vi "check_folder (SubVI).vi"(11 "path in":path) -> (3 "path out":path)   [LabVIEW 2014]
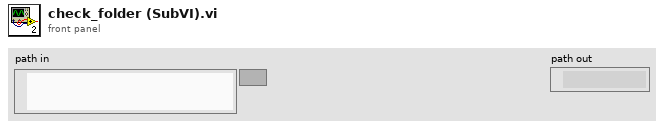
[diagram p1: front panel]
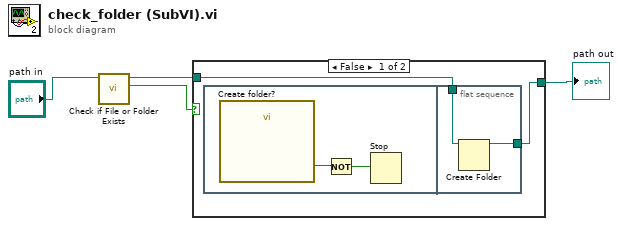
[diagram p0: block diagram]
diagram:
  n1 = call <vilib>:"Check if File or Folder Exists.vi"("path"="path in") -> ("file or folder exists?"=w3:bool, "dup path"=w4:path)  [unwired: 8 in, 1 out]
  n2 = case shown="False" w3 {
    tunnel: w4 -> [w6 w11]
    tunnel: [w5 w11] -> w1
    frame False {
      n3 = flat-sequence {
        tunnel: w6 -> [w10]
        tunnel: [w9] -> w5
        frame #0 {
          n4 = call "Create folder?"() -> ("OK"=w8:bool)  [unwired: 18 in, 1 out]
          n5 = Not(x=w8) -> (.not. x?=w7:bool)
          n6 = Stop(stop? (T)=w7) -> ()
        }
        frame #1 {
          n7 = Create Folder(path (use dialog)=w10) -> (created path=w9:path)  [unwired: 2 in, 2 out]
        }
      }
    }
    frame True {
    }
  }
  "path out" <- w1
